vi "Handle Error.vi"(8 "error in (no error)":errorcluster, 11 "Serial Devices in":refnum<class "Serial Devices.lvclass">) -> (0 "error out":errorcluster, 2 "stop actor?":bool=TRUE, 3 "Serial Devices out":refnum<class "Serial Devices.lvclass">)   [LabVIEW 2019, in "Serial Devices.lvlib" / "Serial Devices.lvclass"]
doc: "(<B>Filename</B>: Actor Framework.lvlib:Actor.lvclass:Handle Error.vi)\n\nDefines how the actor handles an error that occurred while processing a message. By default, this method does nothing except stop the actor."
uses:
  Serial Devices.lvclass
  <vilib>/ActorFramework/Actor/Actor.lvclass
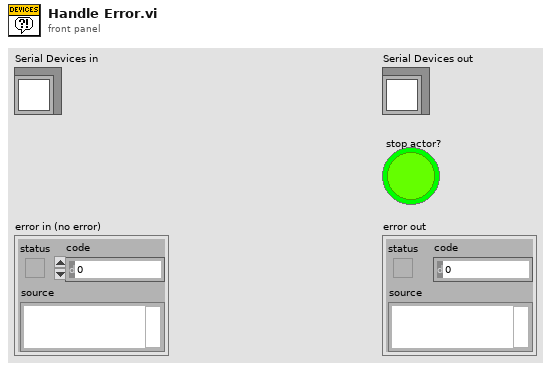
[diagram p1: front panel]
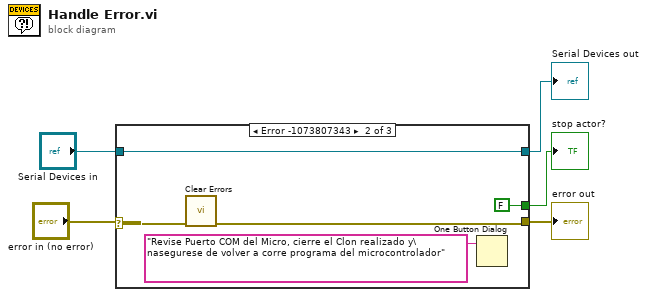
[diagram p0: block diagram]
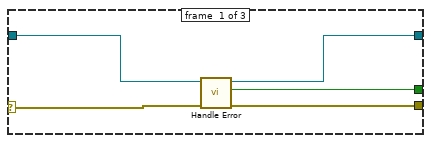
[diagram p2: hidden frame]
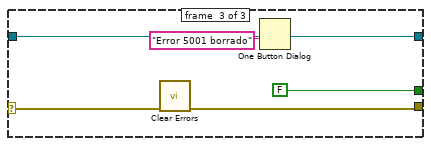
[diagram p3: hidden frame]
diagram:
  n1 = case shown="Error -1073807343" "error in (no error)" {
    selector: "error in (no error)" -> [w6 w15 w20]
    tunnel: [w10 w14 w17] -> w3
    tunnel: [w9 FALSE ("stop actor?") FALSE ("stop actor?")] -> w2
    tunnel: [w8 w12 w16] -> w1
    tunnel: "Serial Devices in" -> [w7 w12 w16]
    frame #0 {
      n2 = call-parent "Handle Error.vi"("error in (no error)"=w6, "Actor in"=w7) -> ("error out"=w10:errorcluster, "stop actor?"=w9:bool, "Actor out"=w8:refnum<class "Serial Devices.lvclass">)  [unwired: 7 in]
    }
    frame #1 {
      n3 = call <vilib>:"Clear Errors.vi"("error in (no error)"=w15) -> ("error out"=w14:errorcluster)  [unwired: 5 in, 1 out]
      n4 = One Button Dialog(message="Revise Puerto COM del Micro, cierre el Clon realizado y\nasegurese de volver a corre programa del microcontrolador") -> ()  [unwired: 1 in, 1 out]
    }
    frame #2 {
      n5 = call <vilib>:"Clear Errors.vi"("error in (no error)"=w20) -> ("error out"=w17:errorcluster)  [unwired: 5 in, 1 out]
      n6 = One Button Dialog(message="Error 5001 borrado") -> ()  [unwired: 1 in, 1 out]
    }
  }
  "Serial Devices out" <- w1
  "error out" <- w3
  "stop actor?" <- w2
